vi "Conditional Disable Helper.vi"   [LabVIEW 2014, in "LMH-LINX.lvlib" / "Local IO.lvlib"]
uses:
  <vilib>/MakerHub/LINX/Private/Local IO/Local IO.lvlib
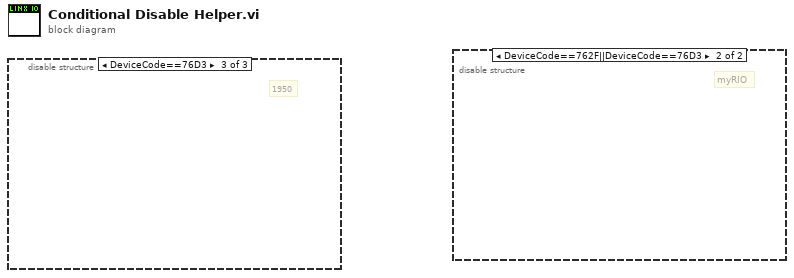
[diagram p0: block diagram]
diagram:
  n1 = disable-structure shown="DeviceCode==76D3" {
    frame condition #0 (active) {
    }
    frame condition #1 {
      # "1900"
    }
    frame condition #2 {
      # "1950"
    }
  }
  n2 = disable-structure shown="DeviceCode==762F||DeviceCode==76D3" {
    frame condition #0 (active) {
    }
    frame condition #1 {
      # "myRIO"
    }
  }
